vi "核查数据断电保存 (子VI).vi"   [LabVIEW 2016, in "数据传输系统.lvlib"]
uses:
  <vilib>/Utility/config.llb/NI_LVConfig.lvlib
types:
  T1 = cluster{"setini":string, "sysini":string, "hechaini":string, "actualwrite":string, "actualread":string, "datasent":string, "反控命令信息队列":string, "反控与仪器交互":string}
  T2 = typedef "NI_LVConfig.lvlib/Config Data RefNum.ctl" = refnum<k1>
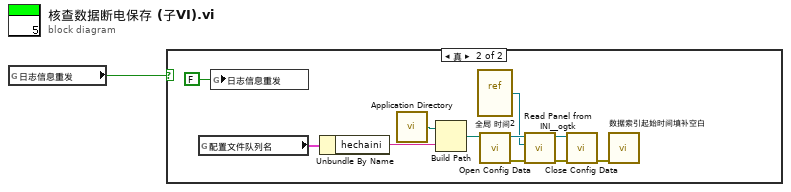
[diagram p0: block diagram]
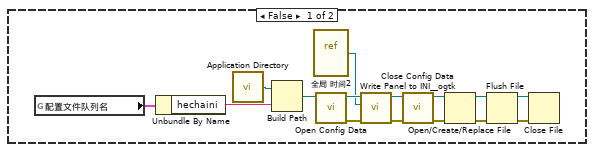
[diagram p2: hidden frame]
diagram:
  n1 = global read "断电保存全局.vi" "日志信息重发"() -> (w1:bool)
  n2 = case shown="真" w1 {
    frame False {
      n3 = global read "断电保存全局.vi" "配置文件队列名"() -> (w3:T1)
      n4 = Unbundle By Name(w3) -> ("hechaini"=w2:string)
      n5 = call <vilib>:"Application Directory.vi"() -> ("Application Directory"=w4:path)
      n6 = Build Path(base path=w4, name or relative path=w2) -> (appended path=w5:path)
      n7 = vi-ref "全局 时间2.vi"() -> (w6:refnum<vi>)
      n8 = call <vilib>:"Open Config Data.vi"("configuration file path"=w5) -> ("error out"=w8:errorcluster, "refnum"=w16:T2)  [unwired: 8 in, 1 out]
      n9 = call <userlib>:"Write Panel to INI__ogtk.vi"("error in (no error)"=w8, "VI ref"=w6, "refnum"=w16) -> ("error out"=w9:errorcluster, "refnum out"=w7:T2)  [unwired: 7 in]
      n10 = call <vilib>:"Close Config Data.vi"("error in (no error)"=w9, "refnum"=w7) -> ("error out"=w14:errorcluster, "file path"=w15:path)  [unwired: 8 in]
      n11 = Open/Create/Replace File(file path (use dialog)=w15, error in=w14) -> (refnum out=w11:refnum<file>, error out=w10:errorcluster)  [unwired: 4 in, 1 out]
      n12 = Flush File(refnum=w11, error in=w10) -> (refnum out=w12:refnum<file>, error out=w13:errorcluster)
      n13 = Close File(refnum=w12, error in=w13) -> ()  [unwired: 2 out]
    }
    frame True {
      n14 = global read "断电保存全局.vi" "配置文件队列名"() -> (w25:T1)
      n15 = global write "断电保存全局.vi" "日志信息重发"(FALSE ("日志信息重发")) -> ()
      n16 = Unbundle By Name(w25) -> ("hechaini"=w26:string)
      n17 = call <vilib>:"Application Directory.vi"() -> ("Application Directory"=w18:path)
      n18 = Build Path(base path=w18, name or relative path=w26) -> (appended path=w17:path)
      n19 = vi-ref "全局 时间2.vi"() -> (w20:refnum<vi>)
      n20 = call <vilib>:"Open Config Data.vi"("configuration file path"=w17) -> ("error out"=w22:errorcluster, "refnum"=w21:T2)  [unwired: 8 in, 1 out]
      n21 = call <userlib>:"Read Panel from INI__ogtk.vi"("error in (no error)"=w22, "VI ref"=w20, "refnum"=w21) -> ("error out"=w23:errorcluster, "refnum out"=w19:T2)  [unwired: 7 in]
      n22 = call <vilib>:"Close Config Data.vi"("error in (no error)"=w23, "refnum"=w19) -> ("error out"=w24:errorcluster)  [unwired: 8 in, 1 out]
      n23 = call "数据索引起始时间填补空白.vi"("error in (no error)"=w24) -> ()  [unwired: 10 in, 1 out]
    }
  }
